vi "sub_save_rawdata.vi"(8 "error in (no error)":errorcluster caption="에러 입력(에러 없음)", 11 "배열":waveform(dbl)[](array[waveform])) -> (0 "error out":errorcluster caption="에러 출력")   [LabVIEW 2013]
uses:
  <vilib>/Waveform/WDTFileIO.llb/ Write Waveforms to File (1D).vi
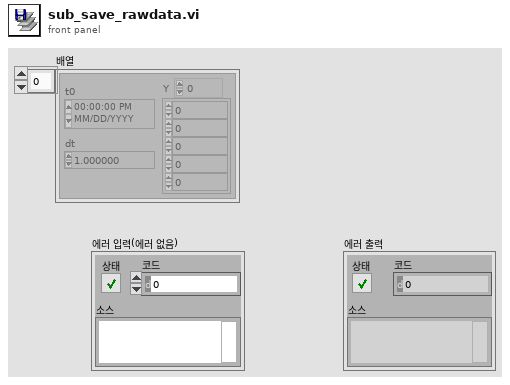
[diagram p1: front panel]
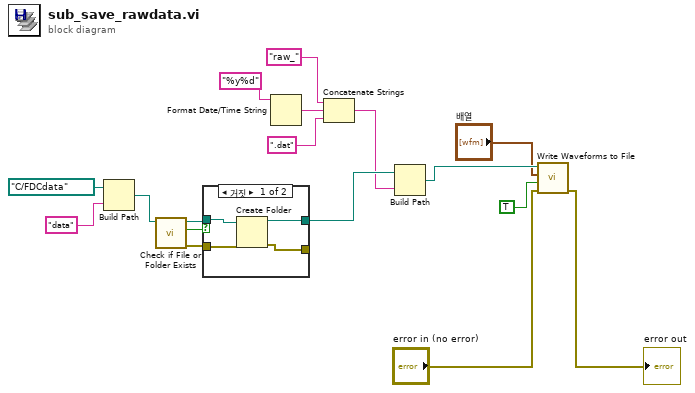
[diagram p0: block diagram]
diagram:
  n1 = Build Path(base path=path "C:/FDCdata" ("베이스 경로"), name or relative path="data" ("이름 또는 상대 경로")) -> (appended path=w11:path)
  n2 = call <vilib>:"Check if File or Folder Exists.vi"("path"=w11) -> ("error out"=w15:errorcluster, "file or folder exists?"=w14:bool, "dup path"=w13:path)  [unwired: 8 in]
  n3 = case shown="거짓" w14 {
    tunnel: w13 -> [w21 w23]
    tunnel: w15 -> [w20 w22]
    tunnel: [w19 w23] -> w10
    tunnel: [w18 w22] -> _
    frame False {
      n4 = Create Folder(path (use dialog)=w21, error in=w20) -> (created path=w19:path, error out=w18:errorcluster)  [unwired: 1 in, 1 out]
    }
    frame True {
    }
  }
  n5 = Format Date/Time String(time format string (%c)="%y%d" ("시간 포맷 문자열 (%c)")) -> (date/time string=w5:string)  [unwired: 2 in]
  n6 = Concatenate Strings("raw_" ("이름 또는 상대 경로"), w5, ".dat" ("문자열")) -> (w7:string)
  n7 = Build Path(base path=w10, name or relative path=w7) -> (appended path=w17:path)
  n8 = call-poly <vilib>:"Write Waveforms to File.vi"("error in (no error)"="error in (no error)", "append to file? (new file:F)"=TRUE, "waveform array"="배열", "file path (dialog if empty)"=w17) -> ("error out"=→"error out":errorcluster)  [unwired: 6 in, 1 out]
